vi "SwerveAccelerationLimiting.vi"(5 "Min Speed Threshold (ft/s)":dbl=5.0 format="%#_13g", 7 "Acceleration Limit (ft/s^2)":dbl=15.0, 8 "Auto Control":bool, 9 "Joystick Y":dbl, 11 "Joystick X":dbl) -> (1 "Limited Joystick Y":dbl, 3 "Limited Joystick X":dbl)   [LabVIEW 2020]
doc: "Limits the acceleration (velocity magnitude and strafe direction change) of the swerve drive. All limits are based on field-relative commands. Ensures that maximum acceleration from a full stop or while pushing against another robot is available."
uses:
  GlobalDrivebase.vi
  GlobalPoseAndTargeting.vi
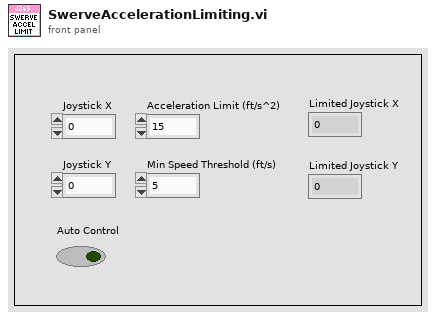
[diagram p1: front panel]
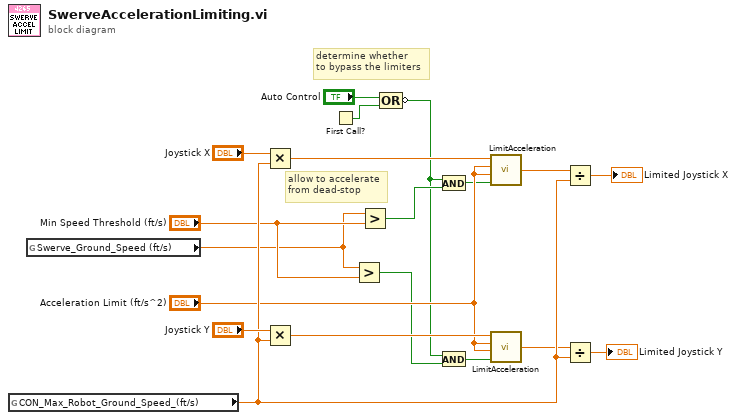
[diagram p0: block diagram]
diagram:
  # "allow to accelerate\nfrom dead-stop"
  # "determine whether \nto bypass the limiters"
  n1 = global read "GlobalDrivebase.vi" "CON_Max_Robot_Ground_Speed_(ft/s)"() -> (w14:dbl)
  n2 = global read "GlobalPoseAndTargeting.vi" "Swerve_Ground_Speed (ft/s)"() -> (w1:dbl)
  n3 = Multiply(x="Joystick X", y=w14) -> (x*y=w18:dbl)
  n4 = Multiply(x="Joystick Y", y=w14) -> (x*y=w17:dbl)
  n5 = First Call?() -> (First Call?: T/F=w8:bool)
  n6 = Greater?(x=w1, y="Min Speed Threshold (ft/s)") -> (0:w3:bool)
  n7 = Greater?(x=w1, y="Min Speed Threshold (ft/s)") -> (0:w5:bool)
  n8 = Compound Arithmetic op=OR("Auto Control", w8) -> (invert w2:bool)
  n9 = And(x=w2, y=w5) -> (x .and. y?=w6:bool)
  n10 = And(x=w2, y=w3) -> (x .and. y?=w4:bool)
  n11 = call "LimitAcceleration.vi"("Apply Limit"=w6, "Decceleration Limit (/s)"="Acceleration Limit (ft/s^2)", "Acceleration Limit (/s)"="Acceleration Limit (ft/s^2)", "Raw Input"=w18) -> ("Output"=w9:dbl)
  n12 = call "LimitAcceleration.vi"("Apply Limit"=w4, "Decceleration Limit (/s)"="Acceleration Limit (ft/s^2)", "Acceleration Limit (/s)"="Acceleration Limit (ft/s^2)", "Raw Input"=w17) -> ("Output"=w10:dbl)
  n13 = Divide(x=w9, y=w14) -> (x/y=→"Limited Joystick X":dbl)
  n14 = Divide(x=w10, y=w14) -> (x/y=→"Limited Joystick Y":dbl)
